vi "GenerateScanArrays.vi"(7 "time stamp":timestamp, 9 "In Trigger Snap Mode?":bool, 10 "Scan Parameters":T1={"Initial Values"=[4.0], "Final Values"=[10.0, 0.0, 0.0], "Step Sizes"=[0.5, 0.0, 0.0], "Parameters to Change"=[enum."6713 Voltage", enum."6713 Voltage", enum."6713 Voltage"], "Channels to Change"=[1, 0, 0], "Number of Parameters to Scan"=1, "Parameter Nickname (no spaces)"=["drop time"], "Scan Base Name"="BlueDetuning_", "Raw_Data Folder"=path "C:/Users/Rydberg/Documents/Data/Raw_Data/84Sr/2014.12.13", "ROI Parameters"={"Background Radius"=0.0, "Atom Radius"=0.0, "X Center"=0.0, "Y Center"=0.0}, "Drop Time (ms)"=1.0, "Phases To Change"=[], "Scan Pulseblaster Channel With Parameter"={"Change PB Time Toggle"=FALSE, "PB Channel"=0.0, "Parameter Number"=0.0}, "Preserve Waveform\nContinuity"=FALSE, "Generated Array Type"=enum."Custom Array From File", "Master Batch Third Column"=0.0, "Master Batch Fourth Column"=0.0, "Master Batch Fifth Column"=0.0, "Current Param. Values"=[81.5, 1.0]} {"Current Param. Values" format="%^#.3e"; "Drop Time (ms)" min=1.0; "Number of Parameters to Scan" min=1}) -> (0 "Parameter Array":dbl[][](array[numeric]), 1 "Array":dbl[](array[numeric]), 2 "Scan Parameters Out":T1={"Initial Values"=[4.0], "Final Values"=[10.0, 0.0, 0.0], "Step Sizes"=[0.5, 0.0, 0.0], "Parameters to Change"=[enum."6713 Voltage", enum."6713 Voltage", enum."6713 Voltage"], "Channels to Change"=[1, 0, 0], "Number of Parameters to Scan"=1, "Parameter Nickname (no spaces)"=["drop time"], "Scan Base Name"="BlueDetuning_", "Raw_Data Folder"=path "C:/Users/Rydberg/Documents/Data/Raw_Data/84Sr/2014.12.13", "ROI Parameters"={"Background Radius"=0.0, "Atom Radius"=0.0, "X Center"=0.0, "Y Center"=0.0}, "Drop Time (ms)"=1.0, "Phases To Change"=[], "Scan Pulseblaster Channel With Parameter"={"Change PB Time Toggle"=FALSE, "PB Channel"=0.0, "Parameter Number"=0.0}, "Preserve Waveform\nContinuity"=FALSE, "Generated Array Type"=enum."Custom Array From File", "Master Batch Third Column"=0.0, "Master Batch Fourth Column"=0.0, "Master Batch Fifth Column"=0.0, "Current Param. Values"=[81.5, 1.0]} {"Current Param. Values" format="%^#.3e"; "Drop Time (ms)" min=1.0; "Number of Parameters to Scan" min=1})   [LabVIEW 2016]
uses:
  Controls/ScanParameters/ScanParametersPanel.ctl
  Controls/ScanParameters/ParameterToChange.ctl
  Controls/ScanParameters/ROI_set.ctl
  Controls/ScanParameters/ScanPBandParam.ctl
  <vilib>/Utility/file.llb/Read From Spreadsheet File (DBL).vi
  <vilib>/Utility/file.llb/Write To Spreadsheet File (DBL).vi
panel:
  out "appended path":path
  # "Select a PB Channel to set with a phase time for evaporation or whatever"
  # "Select a PB Channel to set with a phase time for evaporation or whatever"
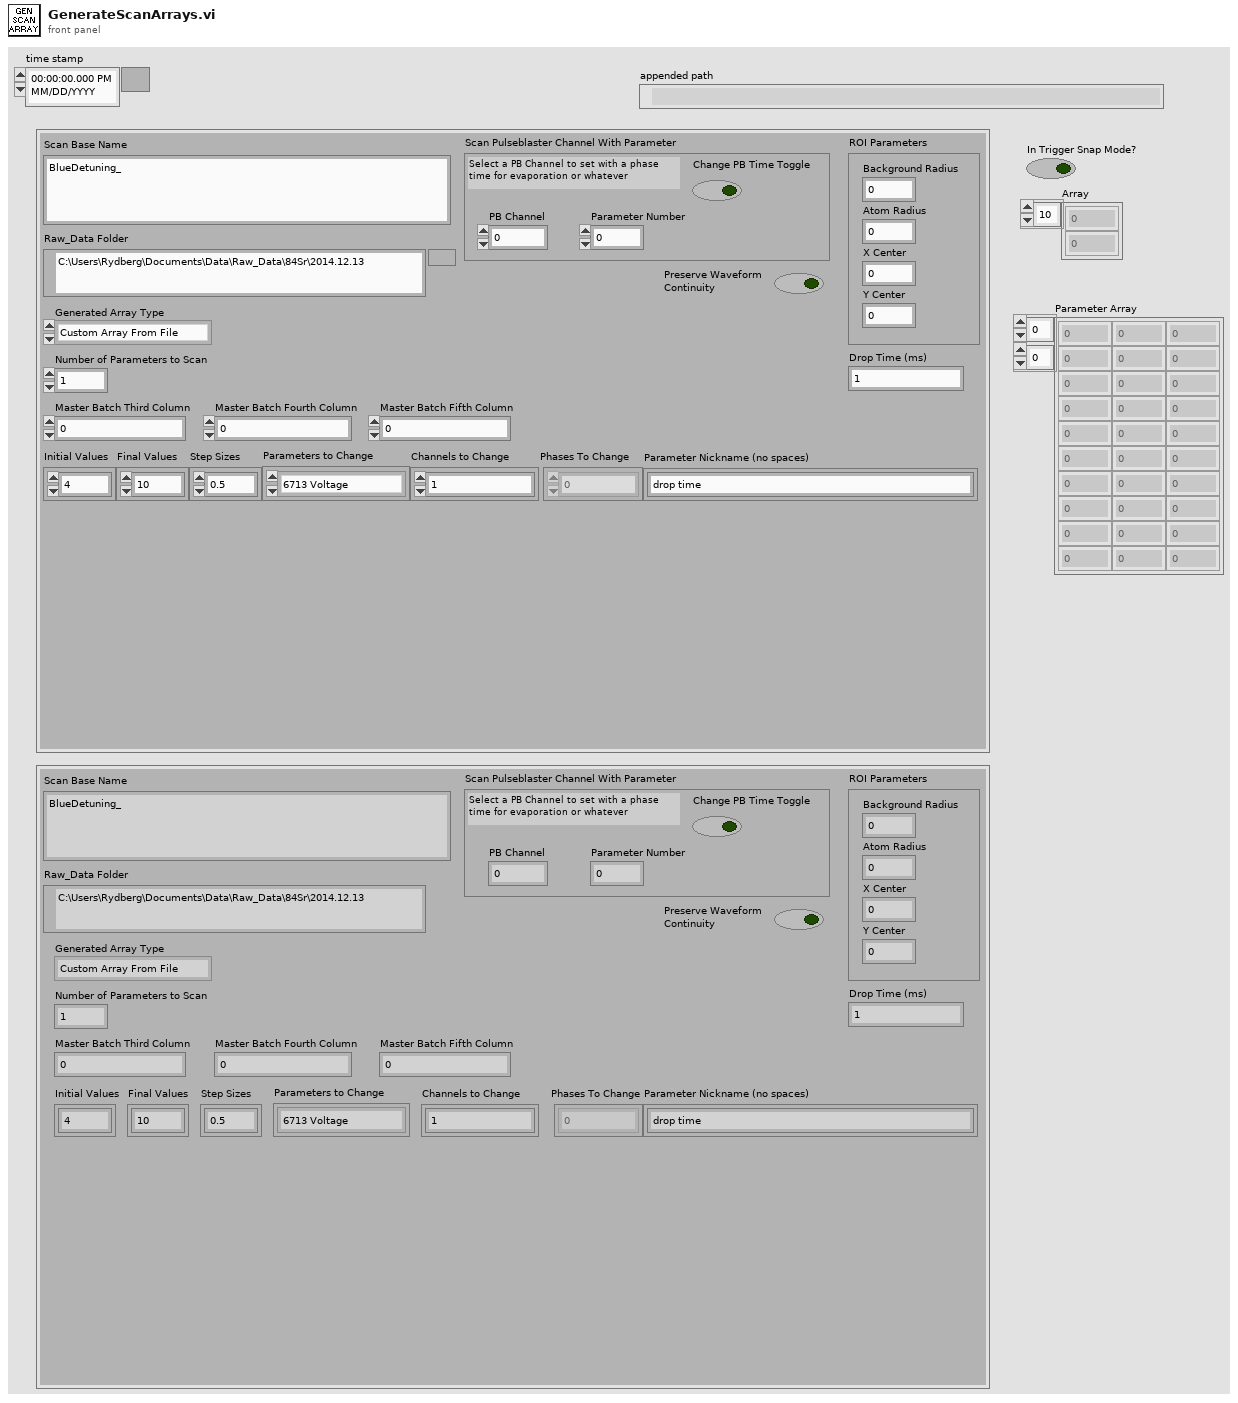
[diagram p1: front panel]
types:
  T1 = typedef "ScanParametersPanel.ctl" = cluster{"Initial Values":dbl[], "Final Values":dbl[], "Step Sizes":dbl[], "Parameters to Change":T2[], "Channels to Change":u32[], "Number of Parameters to Scan":i32, "Parameter Nickname (no spaces)":string[], "Scan Base Name":string, "Raw_Data Folder":path, "ROI Parameters":T3, "Drop Time (ms)":dbl, "Phases To Change":u32[], "Scan Pulseblaster Channel With Parameter":T4, "Preserve Waveform\nContinuity":bool, "Generated Array Type":enum16{"Custom Array From File", "Default (old way)"}, "Master Batch Third Column":dbl, "Master Batch Fourth Column":dbl, "Master Batch Fifth Column":dbl, "Current Param. Values":dbl[]}
  T2 = typedef "ParameterToChange.ctl" = enum16{"Dummy Variable", "Synth Amplitude", "Synth Frequency", "Synth Phase", "ODT Params Phase Time", "ODT Params Tau", "ODT Params Final Voltage", "ODT Params Initial Voltage", "ODT Params Eta", "Red Mot 88 Phase Time", "Red Mot 87 Phase Time", "Red Mot 88 Final Voltage", "Red Mot 88 Initial Voltage", "Red Mot 87 Final Voltage", "Red Mot 87 Initial Voltage", "PulseBlaster", "6713 Voltage", "Green Lattice Phase Time", "Green Lattice Initial Voltage", "Green Lattice Final Voltage", "Agilent Current Setpoint", "FPGA - Constant Op - Set", "FPGA - Bool Op - Output HI", "FPGA - Bool Op - Output LO", "FPGA - Custom Op"}
  T3 = typedef "ROI_set.ctl" = cluster{"Background Radius":dbl, "Atom Radius":dbl, "X Center":dbl, "Y Center":dbl}
  T4 = typedef "ScanPBandParam.ctl" = cluster{"Change PB Time Toggle":bool, "PB Channel":dbl, "Parameter Number":dbl}
  T5 = enum16{"Custom Array From File", "Default (old way)"}
  T6 = enum16{"open", "replace", "create", "open or create", "replace or create", "replace or create with confirmation"}
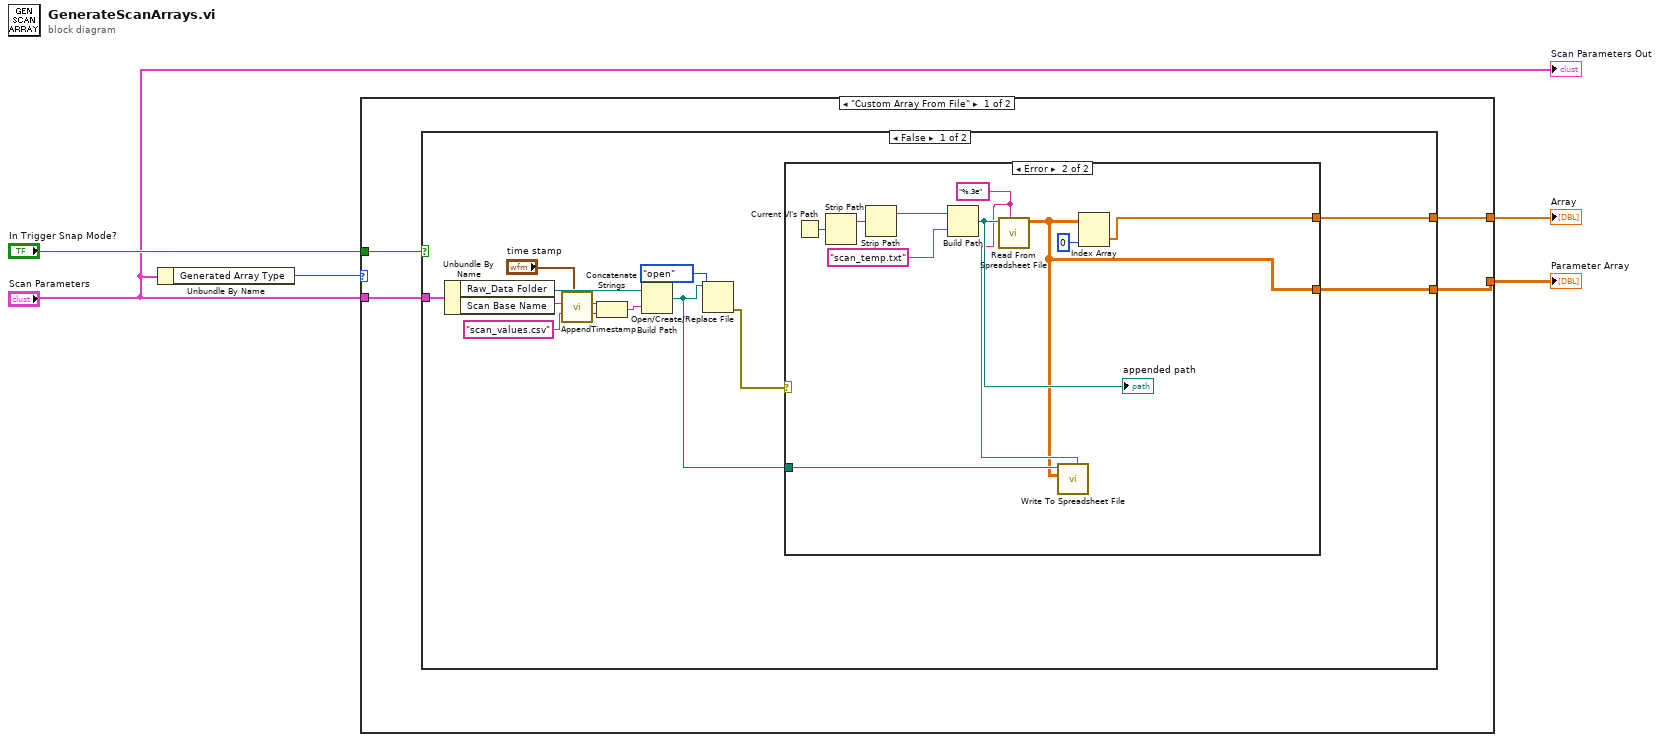
[diagram p0: block diagram]
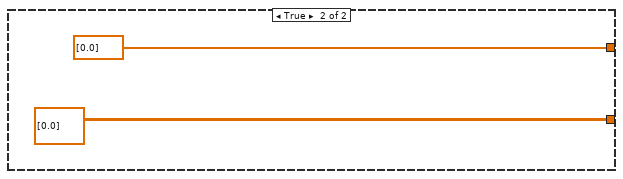
[diagram p3: hidden frame]
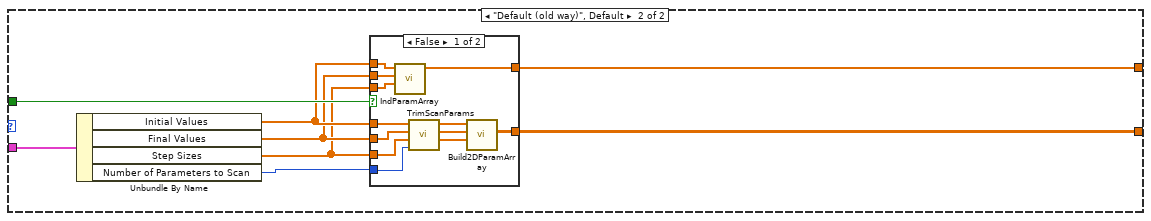
[diagram p4: hidden frame]
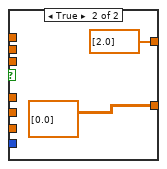
[diagram p5: hidden frame]
diagram:
  n1 = Unbundle By Name("Scan Parameters") -> ("Generated Array Type"=w4:T5)
  n2 = case shown="\"Custom Array From File\"" w4 {
    tunnel: "In Trigger Snap Mode?" -> [w9 w41]
    tunnel: "Scan Parameters" -> [w6 w36]
    tunnel: [w7 w35] -> w2
    tunnel: [w8 w34] -> w1
    frame "Custom Array From File" {
      n3 = case shown="False" w9 {
        tunnel: [w11 dbl[] [0.0] ("Array")] -> w8
        tunnel: [w10 dbl[][] [[0.0]] ("Parameter Array")] -> w7
        tunnel: w6 -> [w21 _]
        frame False {
          n4 = Unbundle By Name(w21) -> ("Raw_Data Folder"=w20:path, "Scan Base Name"=w16:string)
          n5 = call "AppendTimestamp.vi"("time stamp"="time stamp", "String"=w16) -> ("String With Time Added"=w17:string)  [unwired: 9 in]
          n6 = Concatenate Strings(w17, "scan_values.csv" ("string")) -> (w18:string)
          n7 = Build Path(base path=w20, name or relative path=w18) -> (appended path=w12:path)
          n8 = Open/Create/Replace File(file path (use dialog)=w12, operation (0:open)=T6."open") -> (error out=w13:errorcluster)  [unwired: 4 in, 2 out]
          n9 = case shown="Error" w13 {
            tunnel: w12 -> [_ w24]
            tunnel: [_ w25] -> w11
            tunnel: [_ w22] -> w10
            frame No Error {
            }
            frame Error {
              w23 = "%.3e" ("format (%.3f)")
              n10 = Current VI's Path() -> (path=w31:path)
              n11 = Strip Path(path=w31) -> (stripped path=w30:path)  [unwired: 1 out]
              n12 = Strip Path(path=w30) -> (stripped path=w29:path)  [unwired: 1 out]
              n13 = Build Path(base path=w29, name or relative path="scan_temp.txt") -> (appended path=w27:path)
              "appended path" <- w27
              n14 = call-poly <vilib>:"Read From Spreadsheet File.vi"("format (%.3f)"=w23, "file path (dialog if empty)"=w27) -> ("all rows"=w22:dbl[][])  [unwired: 5 in, 4 out]
              n15 = call-poly <vilib>:"Write To Spreadsheet File.vi"("format (%.3f)"=w23, "2D data"=w22, "file path (dialog if empty)"=w24) -> ()  [unwired: 5 in, 1 out]
              n16 = Index Array(array=w22, index (col)=0 ("disabled index (col)")) -> (element=w25:dbl[])  [unwired: 1 in]
            }
          }
        }
        frame True {
        }
      }
    }
    frame "Default (old way)", Default {
      n17 = Unbundle By Name(w36) -> ("Initial Values"=w39:dbl[], "Final Values"=w38:dbl[], "Step Sizes"=w37:dbl[], "Number of Parameters to Scan"=w40:i32)
      n18 = case shown="False" w41 {
        tunnel: w40 -> [w53 _]
        tunnel: w38 -> [w52 _]
        tunnel: w39 -> [w51 _]
        tunnel: [w47 dbl[][] [[0.0]] ("Parameter Array")] -> w35
        tunnel: w39 -> [w46 _]
        tunnel: w38 -> [w45 _]
        tunnel: w37 -> [w44 _]
        tunnel: [w43 dbl[] [2.0] ("Array")] -> w34
        tunnel: w37 -> [w42 _]
        frame False {
          n19 = call "IndParamArray.vi"("Step Sizes"=w44, "Final Values"=w45, "Initial Values"=w46) -> ("Array"=w43:dbl[])  [unwired: 8 in]
          n20 = call "TrimScanParams.vi"("Parameters to change"=w53, "Step Sizes"=w42, "Final Values"=w52, "Initial Values"=w51) -> ("Step Sizes Out"=w48:dbl[], "Final Values Out"=w49:dbl[], "Initial Values Out"=w50:dbl[])  [unwired: 5 in]
          n21 = call "Build2DParamArray.vi"("Step Sizes"=w48, "Final Values"=w49, "Initial Values"=w50) -> ("Parameter Array"=w47:dbl[][])  [unwired: 8 in]
        }
        frame True {
        }
      }
    }
  }
  "Array" <- w1
  "Parameter Array" <- w2
  "Scan Parameters Out" <- "Scan Parameters"
